vi "数据存储.vi"(9 "数据存储标志位":bool, 10 "数据输入":i32[][](array[numeric]), 11 "上一时刻时间":timestamp) -> (1 "初始化缓存":i32[][](array[numeric]), 2 "当前时间":timestamp, 3 "波形图表 6":waveform(i32)[](graph))   [LabVIEW 2020]
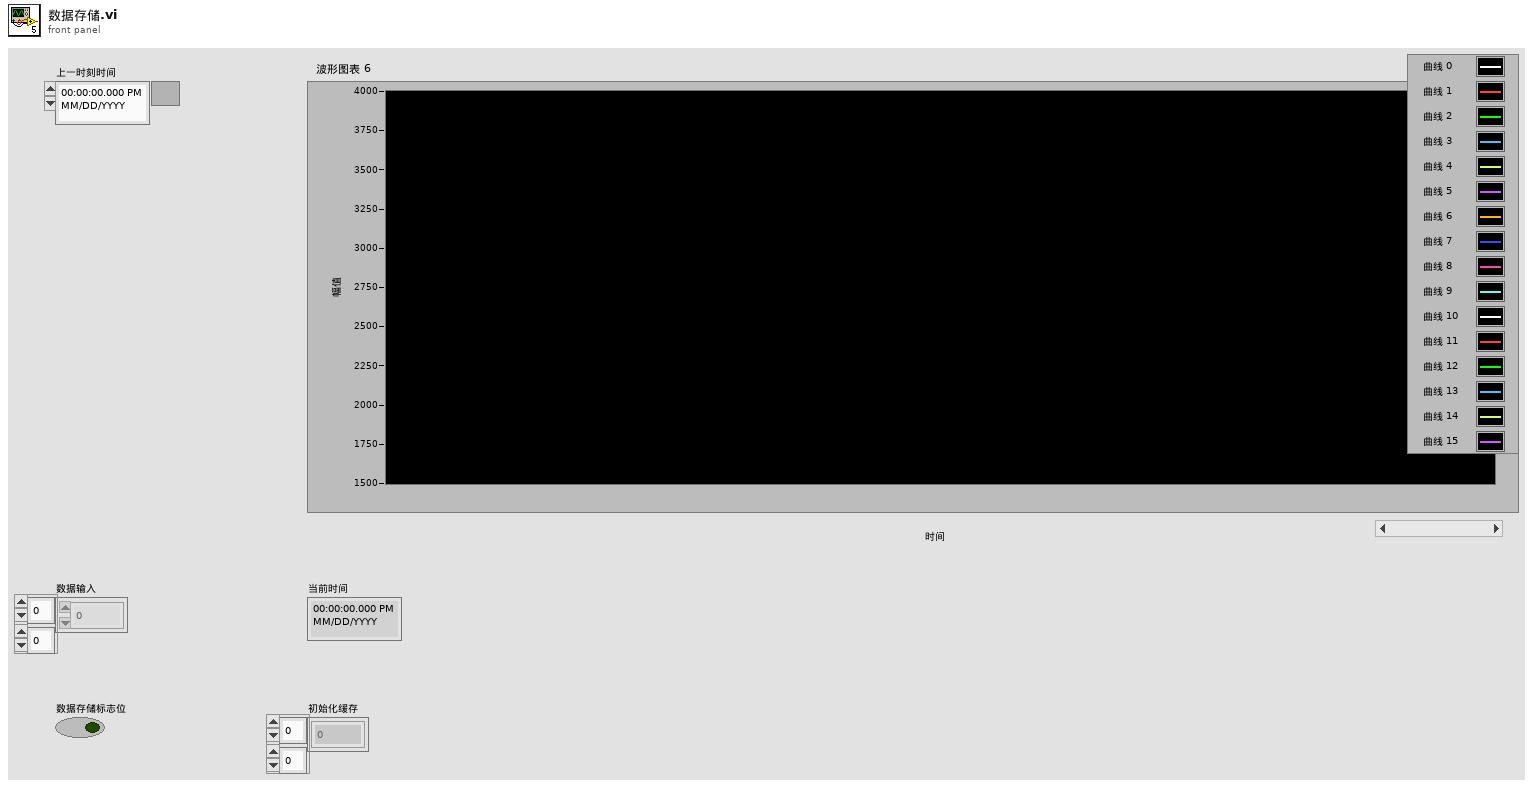
[diagram p1: front panel]
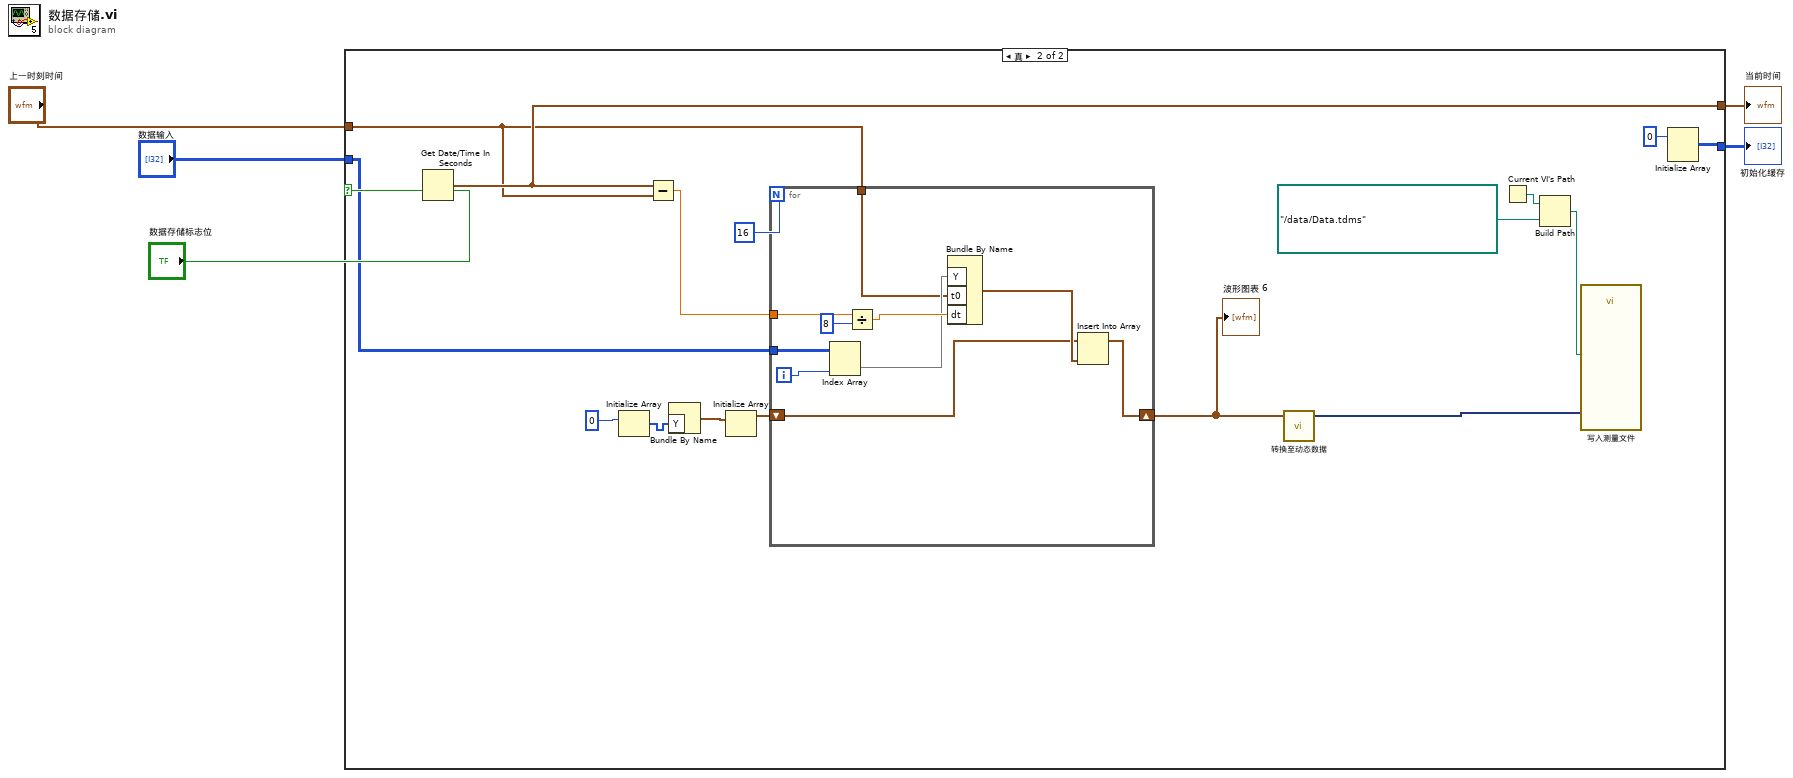
[diagram p0: block diagram]
diagram:
  n1 = case shown="真" "数据存储标志位" {
    tunnel: "数据输入" -> [w7 w13]
    tunnel: [w7 w22] -> w3
    tunnel: [w6 w12] -> w4
    tunnel: "上一时刻时间" -> [w6 w11]
    frame False {
    }
    frame True {
      n2 = Get Date/Time In Seconds() -> (seconds since 1Jan1904=w12:timestamp)
      n3 = Initialize Array(0) -> (w17:i32[])  [unwired: 1 in]
      n4 = Subtract(x=w12, y=w11) -> (x-y=w16:dbl)
      n5 = Bundle By Name ("创建波形")("Y"=w17) -> (w19:waveform(i32))  [unwired: 1 in]
      n6 = Initialize Array(w19) -> (w20:waveform(i32)[])  [unwired: 1 in]
      n7 = for {
        N: 16 -> [_]
        shift-right: [w31] -> w15
        shift-left: w20 -> [w30]
        tunnel: w16 -> [w29]
        tunnel: w13 -> [w26]
        tunnel: w11 -> [w24]
        i -> [w33]
        n8 = Index Array(array=w26, index (col)=w33) -> (element=w25:i32[])  [unwired: 1 in]
        n9 = Divide(x=w29, y=8) -> (x/y=w28:dbl)
        n10 = Bundle By Name ("创建波形")("Y"=w25, "t0"=w24, "dt"=w28) -> (w32:waveform(i32))  [unwired: 1 in]
        n11 = Insert Into Array(array=w30, new element=w32) -> (w31:waveform(i32)[])  [unwired: 1 in]
      }
      "波形图表 6" <- w15
      n12 = call "转换至动态数据"("Array of Waveforms"=w15) -> ("Dynamic Data Type"=w14:dynamicdata)  [unwired: 3 in]
      n13 = Current VI's Path() -> (path=w10:path)
      n14 = Build Path(base path=w10, name or relative path=path "../data/Data.tdms" ("file path")) -> (appended path=w8:path)
      n15 = call "写入测量文件"("Signals"=w14, "Filename"=w8) -> ()  [unwired: 15 in, 3 out]
      n16 = Initialize Array(0) -> (w22:i32[][])  [unwired: 2 in]
    }
  }
  "当前时间" <- w4
  "初始化缓存" <- w3
